vi "Adapt To Type (Core).vi"(7 "Type and Defaults":variant, 8 "error in (no error)":errorcluster, 10 "Variant in":variant, 11 "Nulls as Defaults?":bool) -> (0 "error out":errorcluster, 2 "Variant out":variant)   [LabVIEW 2020, in "openg_variant.lvlib"]
uses:
  openg_variant.lvlib
  Waveform Cluster.ctl
  Empty VCluster Constant.vi
  Null VVariant Constant.vi
  <vilib>/Utility/VariantDataType/VariantType.lvlib
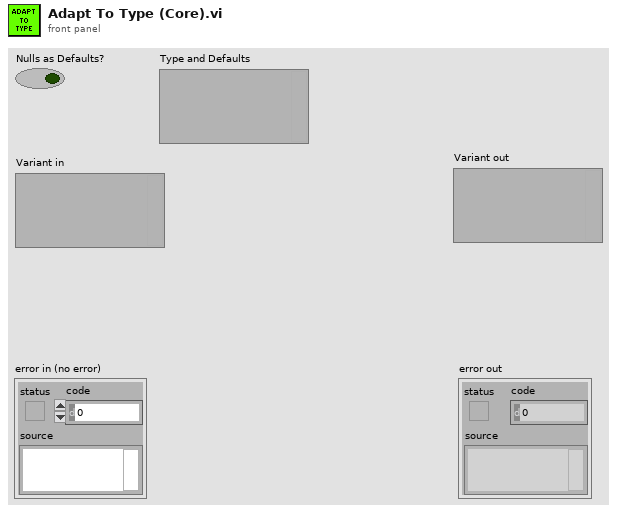
[diagram p1: front panel]
types:
  T1 = typedef "VariantType.lvlib/Type.ctl" = enum8{"Invalid Type", "Void", "I8", "I16", "I32", "I64", "U8", "U16", "U32", "U64", "Single Float", "Double Float", "Extended Float", "Single Complex", "Double Complex", "Extended Complex", "Enum U8", "Enum U16", "Enum U32", "Enum U64", "Single Float With Unit", "Double Float With Unit", "Extended Float With Unit", "Single Complex with Unit", "Double Complex with Unit", "Extended Complex with Unit", "Boolean", "String", "Path", "Picture", "Tag", "Array", "Cluster", "Variant", "LV Variant", "Waveform", "Timestamp", "Digital Waveform", "Digital Data", "ExpressData", "Refnum", "External Data", "VI", "Poly VI", "LabVIEW Class Instance", "Fixed Point"}
  T2 = typedef "openg_variant.lvlib/Waveform Cluster.ctl" = cluster{"t0":timestamp, "dt":dbl, "y":dbl[]}
  T3 = typedef "VariantType.lvlib/MemoryInfo.ctl" = cluster{"Type":T4, "Size":u32}
  T4 = typedef "VariantType.lvlib/MemoryType.ctl" = enum16{"Variable", "Fixed", "Bounded"}
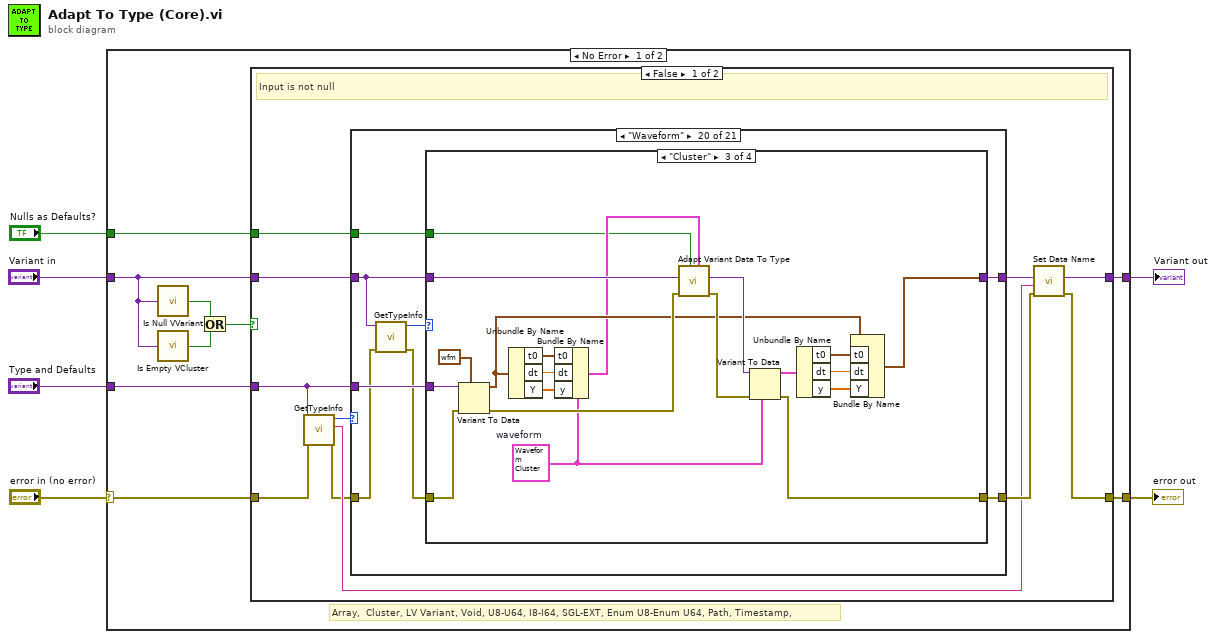
[diagram p0: block diagram]
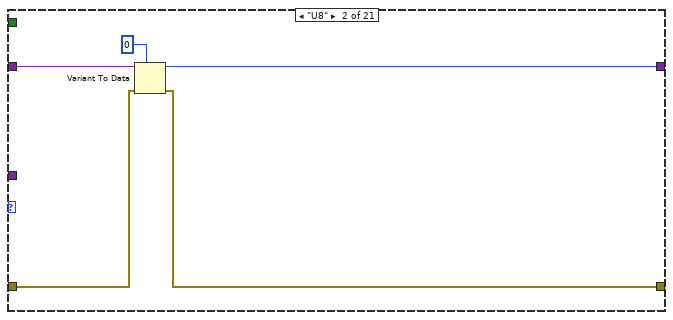
[diagram p3: hidden frame]
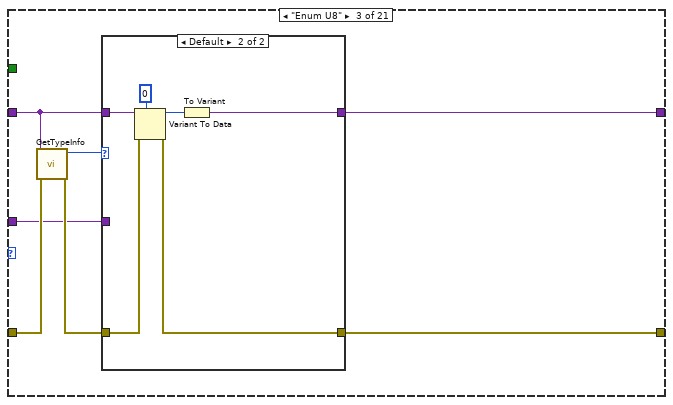
[diagram p4: hidden frame]
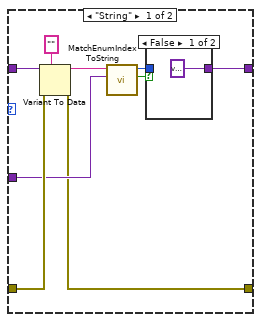
[diagram p5: hidden frame]
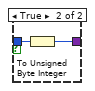
[diagram p6: hidden frame]
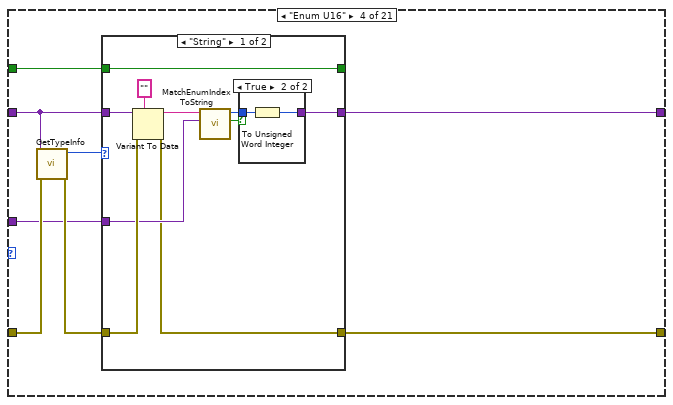
[diagram p7: hidden frame]
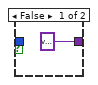
[diagram p8: hidden frame]
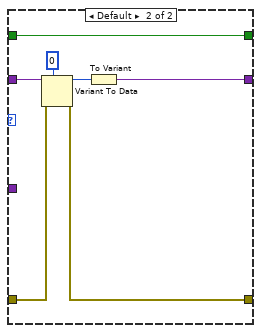
[diagram p9: hidden frame]
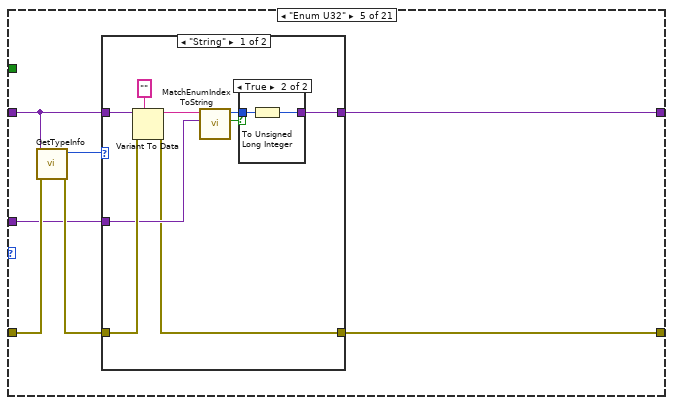
[diagram p10: hidden frame]
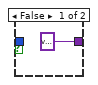
[diagram p11: hidden frame]
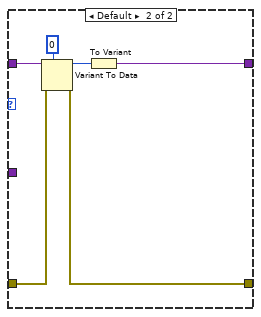
[diagram p12: hidden frame]
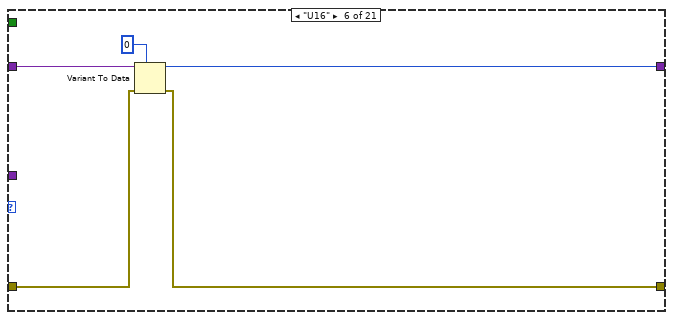
[diagram p13: hidden frame]
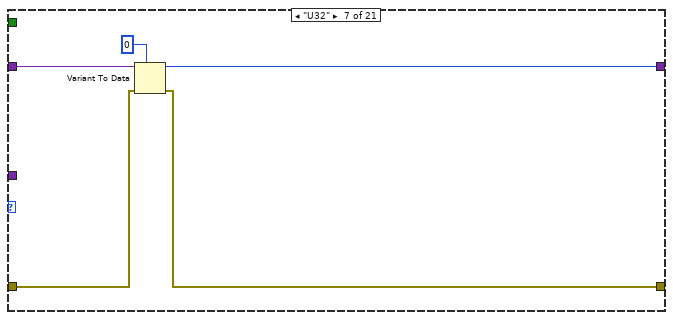
[diagram p14: hidden frame]
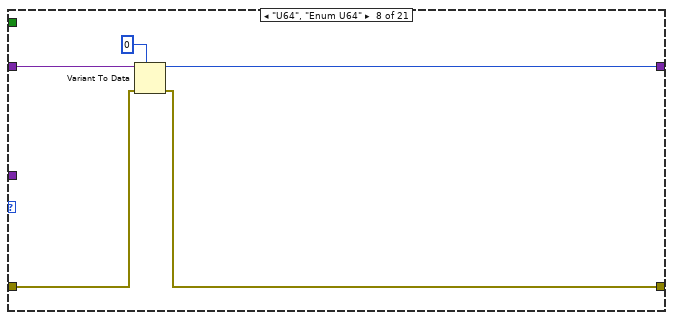
[diagram p15: hidden frame]
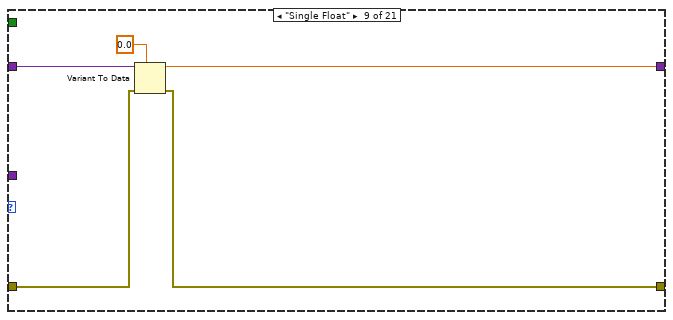
[diagram p16: hidden frame]
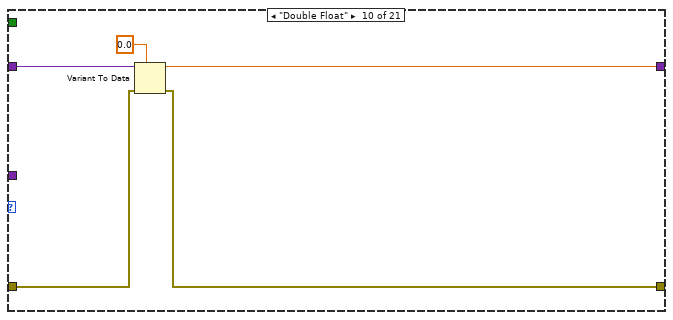
[diagram p17: hidden frame]
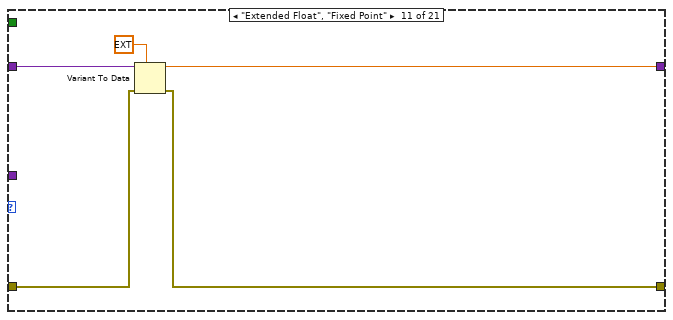
[diagram p18: hidden frame]
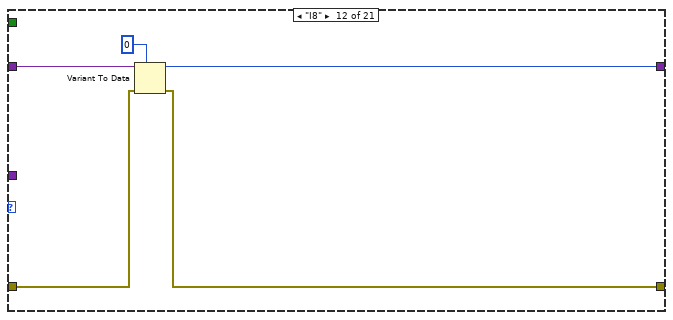
[diagram p19: hidden frame]
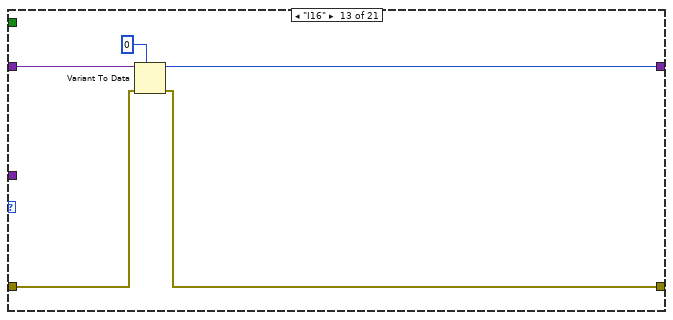
[diagram p20: hidden frame]
diagram:
  n1 = case shown="No Error" "error in (no error)" {
    selector: "error in (no error)" -> [w15 w491]
    tunnel: "Nulls as Defaults?" -> [w7 _]
    tunnel: "Variant in" -> [w11 _]
    tunnel: [w12 w491] -> w3
    tunnel: "Type and Defaults" -> [w14 w490]
    tunnel: [w13 w490] -> w1
    frame No Error {
      # "Array,  Cluster, LV Variant, Void, U8-U64, I8-I64, SGL-EXT, Enum U8-Enum U64, Path, Timestamp,"
      n2 = call "Is Null VVariant.vi"("Variant Data"=w11) -> ("Null?"=w10:bool)
      n3 = call "Is Empty VCluster.vi"("Deserialized JSON Data"=w11) -> ("Empty Cluster?"=w9:bool)
      n4 = Or(x=w10, y=w9) -> (x .or. y?=w8:bool)
      n5 = case shown="False" w8 {
        tunnel: w7 -> [w16 w372]
        tunnel: w15 -> [w25 w374]
        tunnel: w14 -> [w24 w376]
        tunnel: [w22 w377] -> w13
        tunnel: [w21 w373] -> w12
        tunnel: w11 -> [w17 w375]
        frame False {
          # "Input is not null"
          n6 = call <vilib>:"GetTypeInfo.vi"("error in (no error)"=w25, "Variant"=w24) -> ("error out"=w18:errorcluster, "Name"=w19:string, "Type Enum"=w26:T1)  [unwired: 5 in, 2 out]
          n7 = case shown="\"Waveform\"" w26 {
            tunnel: [w28 w31 w38 w64 w91 w114 w119 w124 w129 w134 w139 w144 w149 w154 w159 w167 w169 w180 w251 w325 w370] -> w20
            tunnel: w18 -> [w28 w32 w36 w62 w89 w115 w120 w125 w130 w135 w140 w145 w150 w155 w160 w164 w173 w182 w250 w324 w370]
            tunnel: w16 -> [_ _ _ w60 _ _ _ _ _ _ _ _ _ _ _ _ _ w179 w254 w328 _]
            tunnel: w24 -> [_ _ w34 w59 w87 _ _ _ _ _ _ _ _ _ _ _ _ w183 w253 w327 _]
            tunnel: w17 -> [w27 w33 w39 w65 w92 w116 w121 w126 w131 w136 w141 w146 w151 w156 w161 w165 w174 w175 w248 w322 w371]
            tunnel: [w27 w29 w40 w66 w93 w112 w117 w122 w127 w132 w137 w142 w147 w152 w157 w166 w168 w177 w252 w326 w369] -> w23
            frame "Void", Default {
            }
            frame "U8" {
              n8 = Variant To Data(error in=w32, type=u8 0, Variant=w33) -> (data=w29:u8, error out=w31:errorcluster)
            }
            frame "Enum U8" {
              n9 = call <vilib>:"GetTypeInfo.vi"("error in (no error)"=w36, "Variant"=w39) -> ("error out"=w35:errorcluster, "Type Enum"=w37:T1)  [unwired: 5 in, 3 out]
              n10 = case shown="Default" w37 {
                tunnel: [w43 w53] -> w40
                tunnel: w39 -> [w49 w56]
                tunnel: w35 -> [w47 w55]
                tunnel: [w41 w54] -> w38
                tunnel: w34 -> [w45 _]
                frame "String" {
                  n11 = Variant To Data(error in=w47, type="", Variant=w49) -> (data=w46:string, error out=w41:errorcluster)
                  n12 = call "MatchEnumIndexToString.vi"("Enum Variant"=w45, "String"=w46) -> ("found"=w42:bool, "index"=w44:i32)  [unwired: 8 in]
                  n13 = case shown="False" w42 {
                    tunnel: w44 -> [_ w52]
                    tunnel: [variant ("Type and Defaults") w51] -> w43
                    frame False {
                    }
                    frame True {
                      n14 = To Unsigned Byte Integer(number=w52) -> (unsigned 8bit integer=w51:u8)
                    }
                  }
                }
                frame Default {
                  n15 = Variant To Data(error in=w55, type=u8 0, Variant=w56) -> (data=w57:u8, error out=w54:errorcluster)
                  n16 = To Variant(anything=w57) -> (Variant=w53:variant)
                }
              }
            }
            frame "Enum U16" {
              n17 = call <vilib>:"GetTypeInfo.vi"("error in (no error)"=w62, "Variant"=w65) -> ("error out"=w61:errorcluster, "Type Enum"=w63:T1)  [unwired: 5 in, 3 out]
              n18 = case shown="\"String\"" w63 {
                tunnel: [w70 w80] -> w66
                tunnel: w65 -> [w76 w84]
                tunnel: w61 -> [w74 w83]
                tunnel: [w67 w82] -> w64
                tunnel: w60 -> [w68 w81]
                tunnel: [w68 w81] -> _
                tunnel: w59 -> [w72 _]
                frame "String" {
                  n19 = Variant To Data(error in=w74, type="", Variant=w76) -> (data=w73:string, error out=w67:errorcluster)
                  n20 = call "MatchEnumIndexToString.vi"("Enum Variant"=w72, "String"=w73) -> ("found"=w69:bool, "index"=w71:i32)  [unwired: 8 in]
                  n21 = case shown="True" w69 {
                    tunnel: w71 -> [_ w79]
                    tunnel: [variant ("Type and Defaults") w78] -> w70
                    frame False {
                    }
                    frame True {
                      n22 = To Unsigned Word Integer(number=w79) -> (unsigned 16bit integer=w78:u16)
                    }
                  }
                }
                frame Default {
                  n23 = Variant To Data(error in=w83, type=u16 0, Variant=w84) -> (data=w85:u16, error out=w82:errorcluster)
                  n24 = To Variant(anything=w85) -> (Variant=w80:variant)
                }
              }
            }
            frame "Enum U32" {
              n25 = call <vilib>:"GetTypeInfo.vi"("error in (no error)"=w89, "Variant"=w92) -> ("error out"=w88:errorcluster, "Type Enum"=w90:T1)  [unwired: 5 in, 3 out]
              n26 = case shown="\"String\"" w90 {
                tunnel: [w96 w106] -> w93
                tunnel: w92 -> [w102 w109]
                tunnel: w88 -> [w100 w108]
                tunnel: [w94 w107] -> w91
                tunnel: w87 -> [w98 _]
                frame "String" {
                  n27 = Variant To Data(error in=w100, type="", Variant=w102) -> (data=w99:string, error out=w94:errorcluster)
                  n28 = call "MatchEnumIndexToString.vi"("Enum Variant"=w98, "String"=w99) -> ("found"=w95:bool, "index"=w97:i32)  [unwired: 8 in]
                  n29 = case shown="True" w95 {
                    tunnel: w97 -> [_ w105]
                    tunnel: [variant ("Type and Defaults") w104] -> w96
                    frame False {
                    }
                    frame True {
                      n30 = To Unsigned Long Integer(number=w105) -> (unsigned 32bit integer=w104:u32)
                    }
                  }
                }
                frame Default {
                  n31 = Variant To Data(error in=w108, type=u32 0, Variant=w109) -> (data=w110:u32, error out=w107:errorcluster)
                  n32 = To Variant(anything=w110) -> (Variant=w106:variant)
                }
              }
            }
            frame "U16" {
              n33 = Variant To Data(error in=w115, type=u16 0, Variant=w116) -> (data=w112:u16, error out=w114:errorcluster)
            }
            frame "U32" {
              n34 = Variant To Data(error in=w120, type=u32 0, Variant=w121) -> (data=w117:u32, error out=w119:errorcluster)
            }
            frame "U64", "Enum U64" {
              n35 = Variant To Data(error in=w125, type=u64 0, Variant=w126) -> (data=w122:u64, error out=w124:errorcluster)
            }
            frame "Single Float" {
              n36 = Variant To Data(error in=w130, type=sgl 0.0, Variant=w131) -> (data=w127:sgl, error out=w129:errorcluster)
            }
            frame "Double Float" {
              n37 = Variant To Data(error in=w135, type=0.0, Variant=w136) -> (data=w132:dbl, error out=w134:errorcluster)
            }
            frame "Extended Float", "Fixed Point" {
              n38 = Variant To Data(error in=w140, type=ext 0.0, Variant=w141) -> (data=w137:ext, error out=w139:errorcluster)
            }
            frame "I8" {
              n39 = Variant To Data(error in=w145, type=i8 0, Variant=w146) -> (data=w142:i8, error out=w144:errorcluster)
            }
            frame "I16" {
              n40 = Variant To Data(error in=w150, type=i16 0, Variant=w151) -> (data=w147:i16, error out=w149:errorcluster)
            }
            frame "I32" {
              n41 = Variant To Data(error in=w155, type=0, Variant=w156) -> (data=w152:i32, error out=w154:errorcluster)
            }
            frame "I64" {
              n42 = Variant To Data(error in=w160, type=i64 0, Variant=w161) -> (data=w157:i64, error out=w159:errorcluster)
            }
            frame "Path" {
              n43 = Variant To Data(error in=w164, type="", Variant=w165) -> (data=w162:string, error out=w167:errorcluster)
              n44 = String To Path(string=w162) -> (path=w166:path)
            }
            frame "Timestamp" {
              n45 = Variant To Data(error in=w173, type="", Variant=w174) -> (data=w171:string, error out=w170:errorcluster)
              n46 = call "ISO String To Timestamp.vi"("error in (no error)"=w170, "ISO Timestamp String"=w171) -> ("error out"=w169:errorcluster, "Time Stamp"=w168:timestamp)  [unwired: 8 in]
            }
            frame "Array" {
              n47 = call <vilib>:"GetArrayInfo.vi"("error in (no error)"=w182, "Variant"=w183) -> ("error out"=w181:errorcluster, "ArrayElement"=w178:variant, "NDims"=w176:i32)  [unwired: 6 in, 1 out]
              n48 = case shown="1" w176 {
                tunnel: w181 -> [w186 w192 w231]
                tunnel: w175 -> [w188 w190 w229]
                tunnel: [w187 w196 w235] -> w180
                tunnel: w179 -> [_ w195 w234]
                tunnel: w178 -> [_ w194 w233]
                tunnel: [w188 w193 w232] -> w177
                frame 0, Default {
                  n49 = call <vilib>:"Error Cluster From Error Code.vi"("error in (no error)"=w186, "error message (\"\")"="Unflattening failed. Zero dimensional arrays not supported." ("error message (\"\")"), "error code (0)"=1) -> ("error out"=w187:errorcluster)  [unwired: 6 in]
                }
                frame 1 {
                  n50 = call <vilib>:"GetTypeInfo.vi"("error in (no error)"=w192, "Variant"=w190) -> ("error out"=w191:errorcluster, "Type Enum"=w189:T1)  [unwired: 5 in, 3 out]
                  n51 = case shown="\"Array\"" w189 {
                    tunnel: [w197 w205 w221] -> w196
                    tunnel: w195 -> [_ w199 w220]
                    tunnel: w194 -> [w198 w203 w219]
                    tunnel: [w198 w202 w218] -> w193
                    tunnel: w191 -> [w197 w201 w215]
                    tunnel: w190 -> [_ w200 w217]
                    frame Default {
                    }
                    frame "Array" {
                      n52 = Variant To Data(error in=w201, type=variant[] [], Variant=w200) -> (data=w206:variant[], error out=w204:errorcluster)
                      n53 = for {
                        tunnel: w206 -> [w210] mode=indexing
                        shift-right: [w212] -> w205
                        shift-left: w204 -> [w213]
                        tunnel: w203 -> [w209]
                        tunnel: [w211] -> w202 mode=indexing
                        tunnel: w199 -> [w208]
                        n54 = call "Adapt Variant Data To Type.vi"("Type and Defaults"=w209, "Nulls as Defaults?"=w208, "error in (no error)"=w213, "Variant in"=w210) -> ("error out"=w212:errorcluster, "Variant out"=w211:variant)  [unwired: 6 in]
                      }
                    }
                    frame "Cluster" {
                      n55 = call "Cluster to Array of VData.vi"("error in (no error)"=w215, "Cluster"=w217) -> ("error out"=w216:errorcluster, "Array of VData"=w214:variant[])  [unwired: 8 in]
                      n56 = for {
                        tunnel: w214 -> [w227] mode=indexing
                        shift-right: [w225] -> w221
                        shift-left: w216 -> [w226]
                        tunnel: w219 -> [w223]
                        tunnel: [w224] -> w218 mode=indexing
                        tunnel: w220 -> [w222]
                        n57 = call "Adapt Variant Data To Type.vi"("Type and Defaults"=w223, "Nulls as Defaults?"=w222, "error in (no error)"=w226, "Variant in"=w227) -> ("error out"=w225:errorcluster, "Variant out"=w224:variant)  [unwired: 6 in]
                      }
                    }
                  }
                }
                frame 2.. {
                  n58 = call <vilib>:"GetTypeInfo.vi"("error in (no error)"=w231, "Variant"=w229) -> ("error out"=w230:errorcluster, "Type Enum"=w228:T1)  [unwired: 5 in, 3 out]
                  n59 = case shown="\"Array\"" w228 {
                    tunnel: [w236 w241] -> w235
                    tunnel: w234 -> [_ w238]
                    tunnel: w233 -> [w237 w239]
                    tunnel: [w237 w240] -> w232
                    tunnel: w230 -> [w236 w245]
                    tunnel: w229 -> [_ w244]
                    frame Default {
                    }
                    frame "Array" {
                      n60 = Variant To Data(error in=w245, type=variant[] [], Variant=w244) -> (data=w243:variant[], error out=w242:errorcluster)
                      n61 = call "Hierarchical VArray to MultiD Array.vi"("error in (no error)"=w242, "Element Type"=w239, "Hierarchical Array"=w243, "Nulls as Defaults?"=w238) -> ("error out"=w241:errorcluster, "MultiD Array"=w240:variant)  [unwired: 6 in]
                    }
                  }
                }
              }
            }
            frame "Cluster" {
              n62 = call <vilib>:"GetTypeInfo.vi"("error in (no error)"=w250, "Variant"=w248) -> ("error out"=w249:errorcluster, "Type Enum"=w247:T1)  [unwired: 5 in, 3 out]
              n63 = case shown="\"Cluster\"" w247 {
                tunnel: w254 -> [_ _ w266 w296]
                tunnel: w253 -> [w259 w261 w272 w295]
                tunnel: [w259 w261 w264 w287] -> w252
                tunnel: [w258 w260 w262 w284] -> w251
                tunnel: w249 -> [w257 w260 w271 w283]
                tunnel: w248 -> [_ _ w273 w282]
                frame "Invalid Type", Default {
                  n64 = call <vilib>:"Error Cluster From Error Code.vi"("error in (no error)"=w257, "error message (\"\")"="Cannot deserialize the input type into a cluster." ("error message (\"\")"), "error code (0)"=1) -> ("error out"=w258:errorcluster)  [unwired: 6 in]
                }
                frame "Void" {
                  # "Empty input object, use default values"
                }
                frame "Array" {
                  n65 = call "Cluster to Array of VData.vi"("error in (no error)"=w271, "Cluster"=w272) -> ("error out"=w270:errorcluster, "Array of VData"=w269:variant[])  [unwired: 8 in]
                  n66 = call "Array to Array of VData.vi"("error in (no error)"=w270, "MultiD Array"=w273) -> ("error out"=w267:errorcluster, "1D Array of Variants"=w268:variant[])  [unwired: 8 in]
                  n67 = for {
                    tunnel: w269 -> [w275] mode=indexing
                    tunnel: w268 -> [w281]
                    shift-right: [w277] -> w263
                    shift-left: w267 -> [w278]
                    tunnel: [w276] -> w265 mode=indexing
                    tunnel: w266 -> [w274]
                    i -> [w280]
                    n68 = Index Array(array=w281, index=w280) -> (element=w279:variant)
                    n69 = call "Adapt Variant Data To Type.vi"("Type and Defaults"=w275, "Nulls as Defaults?"=w274, "error in (no error)"=w278, "Variant in"=w279) -> ("error out"=w277:errorcluster, "Variant out"=w276:variant)  [unwired: 6 in]
                  }
                  n70 = call "Array of VData to VCluster.vi"("error in (no error)"=w263, "Array"=w265) -> ("error out"=w262:errorcluster, "VCluster"=w264:variant)  [unwired: 8 in]
                }
                frame "Cluster" {
                  n71 = call "Cluster to Array of VData.vi"("error in (no error)"=w283, "Cluster"=w295) -> ("error out"=w293:errorcluster, "Array of VData"=w294:variant[])  [unwired: 8 in]
                  n72 = call "Cluster to Array of VData.vi"("error in (no error)"=w293, "Cluster"=w282) -> ("error out"=w289:errorcluster, "Array of VData"=w292:variant[])  [unwired: 8 in]
                  n73 = for {
                    tunnel: w292 -> [w298] mode=indexing
                    shift-right: [w299] -> w288
                    shift-left: w289 -> [w300]
                    tunnel: [w298] -> w291 mode=indexing
                    tunnel: [w297] -> w290 mode=indexing
                    n74 = call <vilib>:"GetTypeInfo.vi"("error in (no error)"=w300, "Variant"=w298) -> ("error out"=w299:errorcluster, "Name"=w297:string)  [unwired: 5 in, 3 out]
                  }
                  n75 = for {
                    shift-right: [w309] -> w285
                    shift-left: w288 -> [w305]
                    tunnel: w294 -> [w302] mode=indexing
                    tunnel: [w308] -> w286 mode=indexing
                    tunnel: w291 -> [w303]
                    tunnel: w290 -> [w307]
                    tunnel: w296 -> [w310]
                    n76 = call <vilib>:"GetTypeInfo.vi"("error in (no error)"=w305, "Variant"=w302) -> ("error out"=w304:errorcluster, "Name"=w306:string)  [unwired: 5 in, 3 out]
                    n77 = Search 1D Array(1D array=w307, element=w306) -> (index of element=w301:i32)  [unwired: 1 in]
                    n78 = case shown="0.." w301 {
                      selector: w301 -> [_ w315]
                      tunnel: w310 -> [_ w313]
                      tunnel: [w311 w320] -> w309
                      tunnel: [w312 w319] -> w308
                      tunnel: w304 -> [w311 w318]
                      tunnel: w303 -> [_ w317]
                      tunnel: w302 -> [w312 w314]
                      frame ..-1 {
                        # "Element not found"
                      }
                      frame 0.. {
                        # "Element found"
                        n79 = Index Array(array=w317, index=w315) -> (element=w316:variant)
                        n80 = call "Adapt Variant Data To Type.vi"("Type and Defaults"=w314, "Nulls as Defaults?"=w313, "error in (no error)"=w318, "Variant in"=w316) -> ("error out"=w320:errorcluster, "Variant out"=w319:variant)  [unwired: 6 in]
                      }
                    }
                  }
                  n81 = call "Array of VData to VCluster.vi"("error in (no error)"=w285, "Array"=w286) -> ("error out"=w284:errorcluster, "VCluster"=w287:variant)  [unwired: 8 in]
                }
              }
            }
            frame "Waveform" {
              n82 = call <vilib>:"GetTypeInfo.vi"("error in (no error)"=w324, "Variant"=w322) -> ("error out"=w323:errorcluster, "Type Enum"=w321:T1)  [unwired: 5 in, 3 out]
              n83 = case shown="\"Cluster\"" w321 {
                tunnel: w328 -> [_ _ w336 w356]
                tunnel: w327 -> [w333 w335 w351 w367]
                tunnel: [w333 w335 w338 w359] -> w326
                tunnel: [w332 w334 w339 w360] -> w325
                tunnel: w323 -> [w331 w334 w350 w366]
                tunnel: w322 -> [_ _ w349 w365]
                frame "Invalid Type", Default {
                  n84 = call <vilib>:"Error Cluster From Error Code.vi"("error in (no error)"=w331, "error message (\"\")"="Cannot deserialize the input type into a waveform." ("error message (\"\")"), "error code (0)"=1) -> ("error out"=w332:errorcluster)  [unwired: 6 in]
                }
                frame "Void" {
                  # "Empty input object, use default values"
                }
                frame "Cluster" {
                  w345 = T2 {"t0"=timestamp(0 s since 1904-01-01), "dt"=1.0, "y"=[]}  # waveform
                  n85 = Variant To Data(error in=w350, type=waveform(dbl) {"t0"=timestamp(0 s since 1904-01-01), "dt"=1.0, "Y"=[]}, Variant=w351) -> (data=w344:waveform(dbl), error out=w348:errorcluster)
                  n86 = Unbundle By Name(w344) -> ("t0"=w354:timestamp, "dt"=w353:dbl, "Y"=w352:dbl[])
                  n87 = Bundle By Name(cluster=w345, "t0"=w354, "dt"=w353, "y"=w352) -> (w337:T2)
                  n88 = call "Adapt Variant Data To Type.vi"("Type and Defaults"=w337, "Nulls as Defaults?"=w336, "error in (no error)"=w348, "Variant in"=w349) -> ("error out"=w346:errorcluster, "Variant out"=w347:variant)  [unwired: 6 in]
                  n89 = Variant To Data(error in=w346, type=w345, Variant=w347) -> (data=w343:T2, error out=w339:errorcluster)
                  n90 = Unbundle By Name(w343) -> ("t0"=w342:timestamp, "dt"=w341:dbl, "y"=w340:dbl[])
                  n91 = Bundle By Name(cluster=w344, "t0"=w342, "dt"=w341, "Y"=w340) -> (w338:waveform(dbl))
                }
                frame "Array" {
                  n92 = Variant To Data(error in=w366, type=waveform(dbl) {"t0"=timestamp(0 s since 1904-01-01), "dt"=1.0, "Y"=[]}, Variant=w367) -> (data=w361:waveform(dbl), error out=w364:errorcluster)
                  n93 = Unbundle By Name(w361) -> ("Y"=w357:dbl[])
                  n94 = call "Adapt Variant Data To Type.vi"("Type and Defaults"=w357, "Nulls as Defaults?"=w356, "error in (no error)"=w364, "Variant in"=w365) -> ("error out"=w362:errorcluster, "Variant out"=w363:variant)  [unwired: 6 in]
                  n95 = Variant To Data(error in=w362, type=w357, Variant=w363) -> (data=w358:dbl[], error out=w360:errorcluster)
                  n96 = Bundle By Name(cluster=w361, "Y"=w358) -> (w359:waveform(dbl))
                }
              }
            }
            frame "LV Variant" {
              n97 = To Variant(anything=w371) -> (Variant=w369:variant)
            }
          }
          n98 = call "Set Data Name.vi"("error in (no error)"=w20, "Data Name"=w19, "Data"=w23) -> ("error out"=w21:errorcluster, "Renamed Data"=w22:variant)  [unwired: 7 in]
        }
        frame True {
          # "Input is null"
          n99 = case shown="False" w372 {
            tunnel: [w385 w489] -> w377
            tunnel: w376 -> [w382 w489]
            tunnel: w372 -> [w389 w488]
            tunnel: [w388 w488] -> _
            tunnel: w375 -> [w387 _]
            tunnel: w374 -> [w381 w487]
            tunnel: [w383 w487] -> w373
            frame False {
              # "Return null value if supported by type"
              n100 = call <vilib>:"GetTypeInfo.vi"("error in (no error)"=w381, "Variant"=w382) -> ("error out"=w380:errorcluster, "Name"=w378:string, "Type Enum"=w379:T1)  [unwired: 5 in, 2 out]
              n101 = case shown="\"String\"" w379 {
                tunnel: [w391 w393 w396 w399 w402 w405 w408 w411 w414 w417 w420 w423 w426 w429 w432 w435 w438 w443 w447 w459] -> w384
                tunnel: w380 -> [w391 w393 w396 w399 w402 w405 w408 w411 w414 w417 w420 w423 w426 w429 w432 w435 w438 w443 w450 w461]
                tunnel: w389 -> [w392 w395 w398 w401 w404 w407 w410 w413 w416 w419 w422 w425 w428 w431 w434 w437 w440 w444 w451 w458]
                tunnel: [w392 w395 w398 w401 w404 w407 w410 w413 w416 w419 w422 w425 w428 w431 w434 w437 w440 w444 w451 w456] -> w388
                tunnel: w382 -> [_ _ _ _ _ _ _ _ _ _ _ _ _ _ _ _ _ _ w446 w462]
                tunnel: w387 -> [w390 _ _ _ _ _ _ _ _ _ _ _ _ _ _ _ _ w442 _ w453]
                tunnel: [w390 "" path "" waveform(dbl) {"t0"=timestamp(0 s since 1904-01-01), "dt"=1.0, "Y"=[]} FALSE timestamp(0 s since 1904-01-01) sgl nan nan ext nan u8 0 u16 0 u32 0 u64 0 i8 0 i16 0 0 i64 0 w441 w445 w455] -> w386
                frame "Void", Default {
                }
                frame "String" {
                }
                frame "Path" {
                }
                frame "Waveform" {
                }
                frame "Boolean" {
                }
                frame "Timestamp" {
                }
                frame "Single Float" {
                }
                frame "Double Float" {
                }
                frame "Extended Float", "Fixed Point" {
                }
                frame "U8", "Enum U8" {
                }
                frame "U16", "Enum U16" {
                }
                frame "U32", "Enum U32" {
                }
                frame "U64", "Enum U64" {
                }
                frame "I8" {
                }
                frame "I16" {
                }
                frame "I32" {
                }
                frame "I64" {
                }
                frame "LV Variant" {
                  n102 = To Variant(anything=w442) -> (Variant=w441:variant)
                }
                frame "Cluster" {
                  # "Get cluster default value"
                  n103 = call <vilib>:"GetClusterInfo.vi"("error in (no error)"=w450, "Variant"=w446) -> ("error out"=w448:errorcluster, "Cluster Elements"=w449:variant[])  [unwired: 8 in]
                  n104 = call <vilib>:"SetClusterInfo.vi"("error in (no error)"=w448, "Cluster Elements"=w449, "Variant"=w446) -> ("error out"=w447:errorcluster, "Variant Out"=w445:variant)  [unwired: 7 in]
                }
                frame "Array" {
                  n105 = call <vilib>:"GetArrayInfo.vi"("error in (no error)"=w461, "Variant"=w462) -> ("error out"=w460:errorcluster, "ArrayElement"=w457:variant, "Array Lengths"=w452:T3[], "NDims"=w454:i32)  [unwired: 6 in]
                  n106 = case shown="1" w454 {
                    tunnel: w460 -> [w465 w472 w485]
                    tunnel: w453 -> [w467 _ _]
                    tunnel: [w466 w469 w479] -> w459
                    tunnel: w458 -> [w468 w473 w486]
                    tunnel: w457 -> [_ w471 w484]
                    tunnel: [w468 w473 w486] -> w456
                    tunnel: [w467 w474 w481] -> w455
                    tunnel: w452 -> [_ _ w478]
                    frame 0, Default {
                      n107 = call <vilib>:"Error Cluster From Error Code.vi"("error in (no error)"=w465, "error message (\"\")"="Unflattening failed. Zero dimensional arrays not supported." ("error message (\"\")"), "error code (0)"=1) -> ("error out"=w466:errorcluster)  [unwired: 6 in]
                    }
                    frame 1 {
                      n108 = call "Array of VData to VArray.vi"("error in (no error)"=w472, "Element Type (when empty)"=w471, "1D Array of VData"=variant[] []) -> ("error out"=w469:errorcluster, "VArray"=w474:variant)  [unwired: 7 in]
                    }
                    frame 2.. {
                      n109 = Array Size(array=w478) -> (size(s)=w477:i32)
                      n110 = Initialize Array(0, w477) -> (w475:i32[])
                      n111 = call "Array of VData to VArray.vi"("error in (no error)"=w485, "Element Type (when empty)"=w484, "1D Array of VData"=variant[] []) -> ("error out"=w480:errorcluster, "VArray"=w482:variant)  [unwired: 7 in]
                      n112 = call "Reshape 1D Array.vi"("error in (no error)"=w480, "Size(s)"=w475, "1D Array"=w482) -> ("error out"=w479:errorcluster, "Reshaped VArray"=w481:variant)  [unwired: 7 in]
                    }
                  }
                }
              }
              n113 = call "Set Data Name.vi"("error in (no error)"=w384, "Data Name"=w378, "Data"=w386) -> ("error out"=w383:errorcluster, "Renamed Data"=w385:variant)  [unwired: 7 in]
            }
            frame True {
              # "Return default value"
            }
          }
        }
      }
    }
    frame Error {
    }
  }
  "error out" <- w3
  "Variant out" <- w1
